vi "Untitled 1 (SubVI).vi"(8 "error in (no error)":errorcluster, 9 "Temp and Field Range in":T1, 10 "ACK Q":refnum<queue>, 11 "Queue in":refnum<queue>) -> (0 "error out":errorcluster, 2 "Temp and Field Range out":T1, 3 "Queue out":refnum<queue>)   [LabVIEW 2025]
uses:
  Mag & Temp STM/CTLS/Sweeper.ctl
  Mag & Temp STM/CTLS/ACK.ctl
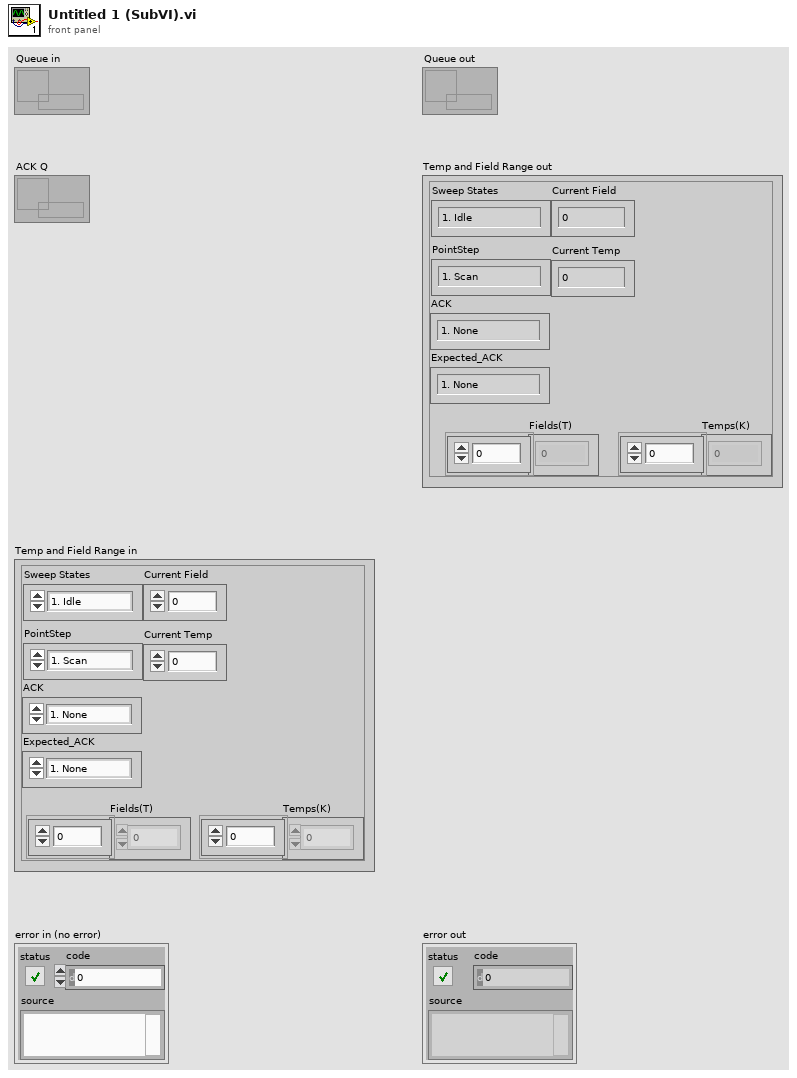
[diagram p1: front panel]
types:
  T1 = typedef "Sweeper.ctl" = cluster{"Temps(K)":dbl[], "Fields(T)":dbl[], "Sweep States":enum16{"1. Idle", "2. Start", "3. Stop", "4. Wait ACK", "5. Bias", "6. Scan", "7. Change Field", "8. Chang Temp", "9. Drift Correct (SF)", "10. Drift Correct (BS)", "11. Next Field", "12. Next Temp"}, "PointStep":enum16{"1. Scan", "2. Drift Correct (SF) #1", "3. Drift Correct (BS) #1", "4. Bias", "5. Scan", "6. Drift Correct (SF) #2", "7. Drift Correct (BS) #2", "8. Done"}, "Current Field":dbl, "Current Temp":dbl, "Expected_ACK":enum16{"1. None", "2. TempStable", "3. FieldStable", "4. ConfigApplied", "5. ScanDone", "6. BiasDone", "7. DriftDone (SF)", "8. DrifDone (BS)", "9. Done"}, "ACK":enum16{"1. None", "2. TempStable", "3. FieldStable", "4. ConfigApplied", "5. ScanDone", "6. BiasDone", "7. DriftDone (SF)", "8. DrifDone (BS)", "9. Done"}}
  T2 = typedef "ACK.ctl" = cluster{"ACK":enum16{"1. None", "2. TempStable", "3. FieldStable", "4. ConfigApplied", "5. ScanDone", "6. BiasDone", "7. DriftDone (SF)", "8. DrifDone (BS)"}}
  T3 = enum16{"1. None", "2. TempStable", "3. FieldStable", "4. ConfigApplied", "5. ScanDone", "6. BiasDone", "7. DriftDone (SF)", "8. DrifDone (BS)", "9. Done"}
  T4 = enum16{"1. None", "2. TempStable", "3. FieldStable", "4. ConfigApplied", "5. ScanDone", "6. BiasDone", "7. DriftDone (SF)", "8. DrifDone (BS)"}
  T5 = enum16{"1. Idle", "2. Start", "3. Stop", "4. Wait ACK", "5. Bias", "6. Scan", "7. Change Field", "8. Chang Temp", "9. Drift Correct (SF)", "10. Drift Correct (BS)", "11. Next Field", "12. Next Temp"}
  T6 = enum16{"1. Scan", "2. Drift Correct (SF) #1", "3. Drift Correct (BS) #1", "4. Bias", "5. Scan", "6. Drift Correct (SF) #2", "7. Drift Correct (BS) #2", "8. Done"}
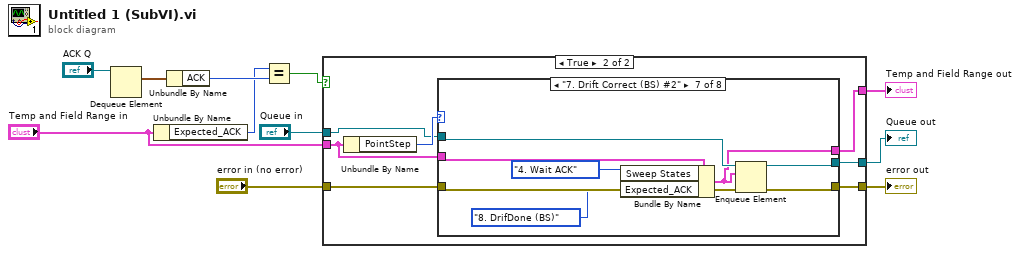
[diagram p0: block diagram]
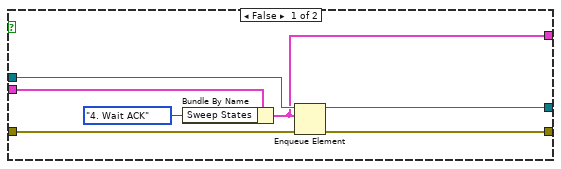
[diagram p2: hidden frame]
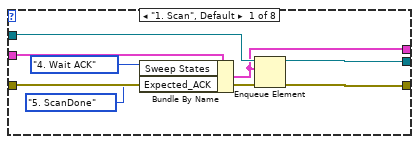
[diagram p3: hidden frame]
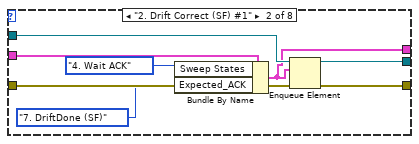
[diagram p4: hidden frame]
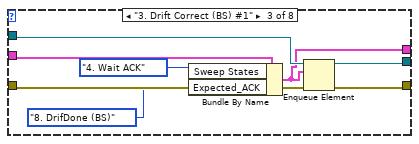
[diagram p5: hidden frame]
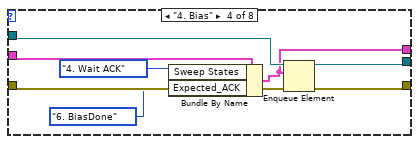
[diagram p6: hidden frame]
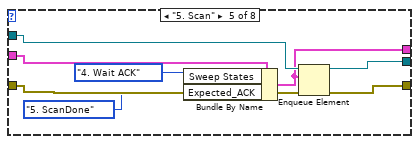
[diagram p7: hidden frame]
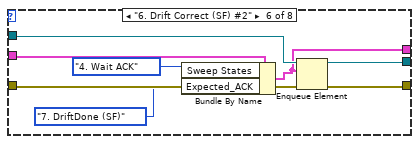
[diagram p8: hidden frame]
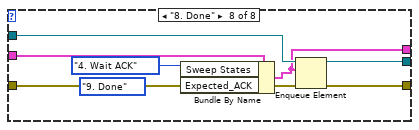
[diagram p9: hidden frame]
diagram:
  n1 = Dequeue Element(queue="ACK Q") -> (element=w2:T2)  [unwired: 2 in, 3 out]
  n2 = Unbundle By Name("Temp and Field Range in") -> ("Expected_ACK"=w3:T3)
  n3 = Unbundle By Name(w2) -> ("ACK"=w4:T4)
  n4 = Equal?(x=w3, y=w4) -> (x = y?=w5:bool)
  n5 = case shown="True" w5 {
    tunnel: "Queue in" -> [w18 w24]
    tunnel: "Temp and Field Range in" -> [w17 w23]
    tunnel: [w15 w22] -> w8
    tunnel: [w14 w21] -> w9
    tunnel: "error in (no error)" -> [w13 w20]
    tunnel: [w12 w19] -> w11
    frame False {
      n6 = Bundle By Name(cluster=w17, "Sweep States"=T5."4. Wait ACK") -> (w12:T1)
      n7 = Enqueue Element(queue=w18, element=w12, error in (no error)=w13) -> (queue out=w15:refnum<queue>, error out=w14:errorcluster)  [unwired: 1 in, 1 out]
    }
    frame True {
      n8 = Unbundle By Name(w23) -> ("PointStep"=w25:T6)
      n9 = case shown="\"7. Drift Correct (BS) #2\"" w25 {
        tunnel: w24 -> [w33 w40 w48 w56 w64 w72 w80 w88]
        tunnel: w23 -> [w32 w39 w47 w55 w63 w71 w79 w87]
        tunnel: [w31 w37 w45 w53 w61 w69 w77 w85] -> w22
        tunnel: [w30 w36 w44 w52 w60 w67 w76 w84] -> w21
        tunnel: w20 -> [w29 w38 w46 w54 w62 w70 w78 w86]
        tunnel: [w28 w35 w43 w51 w59 w68 w75 w83] -> w19
        frame "1. Scan", Default {
          n10 = Bundle By Name(cluster=w32, "Sweep States"=T5."4. Wait ACK", "Expected_ACK"=T3."5. ScanDone") -> (w28:T1)
          n11 = Enqueue Element(queue=w33, element=w28, error in (no error)=w29) -> (queue out=w31:refnum<queue>, error out=w30:errorcluster)  [unwired: 1 in, 1 out]
        }
        frame "2. Drift Correct (SF) #1" {
          n12 = Bundle By Name(cluster=w39, "Sweep States"=T5."4. Wait ACK", "Expected_ACK"=T3."7. DriftDone (SF)") -> (w35:T1)
          n13 = Enqueue Element(queue=w40, element=w35, error in (no error)=w38) -> (queue out=w37:refnum<queue>, error out=w36:errorcluster)  [unwired: 1 in, 1 out]
        }
        frame "3. Drift Correct (BS) #1" {
          n14 = Bundle By Name(cluster=w47, "Sweep States"=T5."4. Wait ACK", "Expected_ACK"=T3."8. DrifDone (BS)") -> (w43:T1)
          n15 = Enqueue Element(queue=w48, element=w43, error in (no error)=w46) -> (queue out=w45:refnum<queue>, error out=w44:errorcluster)  [unwired: 1 in, 1 out]
        }
        frame "4. Bias" {
          n16 = Bundle By Name(cluster=w55, "Sweep States"=T5."4. Wait ACK", "Expected_ACK"=T3."6. BiasDone") -> (w51:T1)
          n17 = Enqueue Element(queue=w56, element=w51, error in (no error)=w54) -> (queue out=w53:refnum<queue>, error out=w52:errorcluster)  [unwired: 1 in, 1 out]
        }
        frame "5. Scan" {
          n18 = Bundle By Name(cluster=w63, "Sweep States"=T5."4. Wait ACK", "Expected_ACK"=T3."5. ScanDone") -> (w59:T1)
          n19 = Enqueue Element(queue=w64, element=w59, error in (no error)=w62) -> (queue out=w61:refnum<queue>, error out=w60:errorcluster)  [unwired: 1 in, 1 out]
        }
        frame "6. Drift Correct (SF) #2" {
          n20 = Bundle By Name(cluster=w71, "Sweep States"=T5."4. Wait ACK", "Expected_ACK"=T3."7. DriftDone (SF)") -> (w68:T1)
          n21 = Enqueue Element(queue=w72, element=w68, error in (no error)=w70) -> (queue out=w69:refnum<queue>, error out=w67:errorcluster)  [unwired: 1 in, 1 out]
        }
        frame "7. Drift Correct (BS) #2" {
          n22 = Bundle By Name(cluster=w79, "Sweep States"=T5."4. Wait ACK", "Expected_ACK"=T3."8. DrifDone (BS)") -> (w75:T1)
          n23 = Enqueue Element(queue=w80, element=w75, error in (no error)=w78) -> (queue out=w77:refnum<queue>, error out=w76:errorcluster)  [unwired: 1 in, 1 out]
        }
        frame "8. Done" {
          n24 = Bundle By Name(cluster=w87, "Sweep States"=T5."4. Wait ACK", "Expected_ACK"=T3."9. Done") -> (w83:T1)
          n25 = Enqueue Element(queue=w88, element=w83, error in (no error)=w86) -> (queue out=w85:refnum<queue>, error out=w84:errorcluster)  [unwired: 1 in, 1 out]
        }
      }
    }
  }
  "Temp and Field Range out" <- w11
  "error out" <- w9
  "Queue out" <- w8
